vi "Calculate Bundle Module Message AutoToolRegion.vi"(1 "Bounds":T1, 2 "Terms":T3) -> (0 "Regions":cluster{"Bounds":T7, "Autotool":T10}[](array[cluster]))   [LabVIEW 2025]
uses:
  <vilib>/XNodeSupport/XNodeRect32.ctl
  <vilib>/XNodeSupport/XNodeInt.ctl
  <vilib>/XNodeSupport/XNodeTools.ctl
  <vilib>/XNodeSupport/XNodeTerm4Array.ctl
  <vilib>/XNodeSupport/XNodeTerm4.ctl
  <vilib>/XNodeSupport/XNodeString.ctl
  <vilib>/XNodeSupport/XNodeVariant.ctl
  <vilib>/XNodeSupport/XNodeBool.ctl
  <vilib>/XNodeSupport/XNodeTermDirection.ctl
  <vilib>/XNodeSupport/XNodeBounds.ctl
  <vilib>/XNodeSupport/NI_XNodeSupport.lvlib
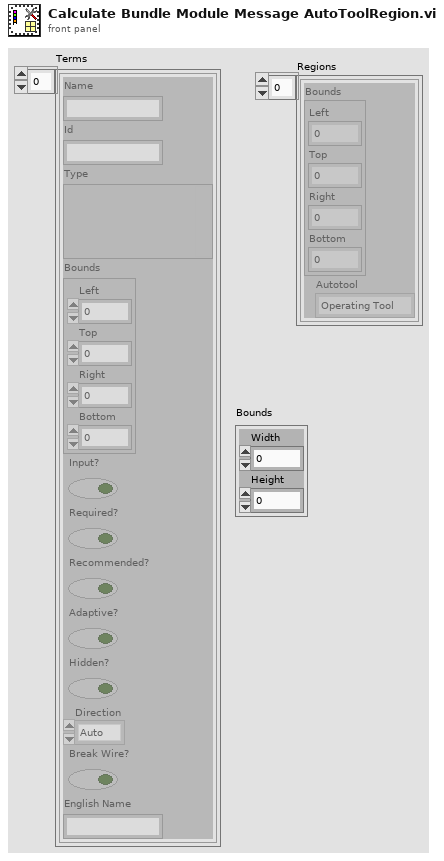
[diagram p1: front panel]
types:
  T1 = typedef "NI_XNodeSupport.lvlib/XNodeBounds.ctl" = cluster{"Width":T2, "Height":T2}
  T2 = typedef "NI_XNodeSupport.lvlib/XNodeInt.ctl" = i32
  T3 = typedef "NI_XNodeSupport.lvlib/XNodeTerm4Array.ctl" = T4[]
  T4 = typedef "NI_XNodeSupport.lvlib/XNodeTerm4.ctl" = cluster{"Name":T5, "Id":T5, "Type":T6, "Bounds":T7, "Input?":T8, "Required?":T8, "Recommended?":T8, "Adaptive?":T8, "Hidden?":T8, "Direction":T9, "Break Wire?":T8, "English Name":T5}
  T5 = typedef "NI_XNodeSupport.lvlib/XNodeString.ctl" = string
  T6 = typedef "NI_XNodeSupport.lvlib/XNodeVariant.ctl" = variant
  T7 = typedef "NI_XNodeSupport.lvlib/XNodeRect32.ctl" = cluster{"Left":T2, "Top":T2, "Right":T2, "Bottom":T2}
  T8 = typedef "NI_XNodeSupport.lvlib/XNodeBool.ctl" = bool
  T9 = typedef "NI_XNodeSupport.lvlib/XNodeTermDirection.ctl" = enum32{"Auto", "Up", "Down", "Left", "Right", "Center"}
  T10 = typedef "NI_XNodeSupport.lvlib/XNodeTools.ctl" = enum32{"Operating Tool", "Placement Tool", "Labelling Tool", "Wiring Tool", "Scroll Tool", "Breakpoint Tool", "Probe Tool", "Auto Tool"}
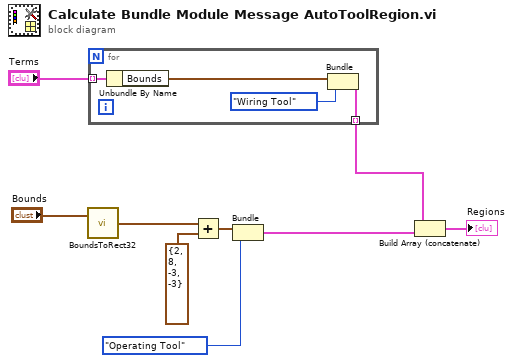
[diagram p0: block diagram]
diagram:
  n1 = call <vilib>:"BoundsToRect32.vi"("Bounds"="Bounds") -> ("Rect32"=w5:T7)  [unwired: 1 in]
  n2 = for {
    tunnel: "Terms" -> [w13] mode=indexing
    tunnel: [w10] -> w4 mode=indexing
    n3 = Unbundle By Name(w13) -> ("Bounds"=w12:T7)
    n4 = Bundle("Bounds"=w12, "Autotool"=XNodeTools."Wiring Tool") -> (w10:cluster{"Bounds":T7, "Autotool":T10})  [unwired: 1 in]
  }
  n5 = Add(x=w5, y=T7 {"Left"=2, "Top"=8, "Right"=-3, "Bottom"=-3}) -> (x+y=w2:T7)
  n6 = Bundle("Rect32"=w2, "Autotool"=XNodeTools."Operating Tool") -> (w7:cluster{"Rect32":T7, "Autotool":T10})  [unwired: 1 in]
  n7 = Build Array (concatenate)(w4, w7) -> (→"Regions":cluster{"Rect32":T7, "Autotool":T10}[])
